vi "FirstRunTest.vi"(11 "Array":string[](array[string])) -> (2 "Message to log to console":string, 3 "exit code":i32)   [LabVIEW 2018]
uses:
  <vilib>/Utility/error.llb/DialogType.ctl
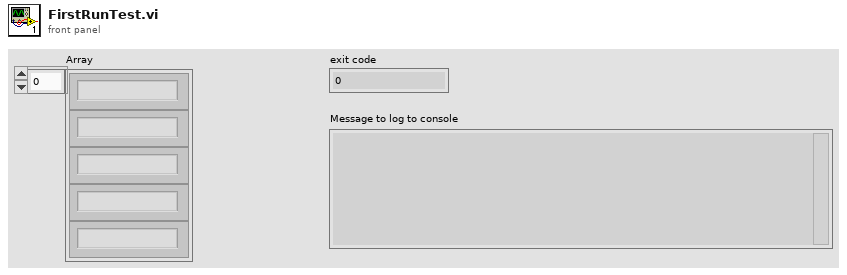
[diagram p1: front panel]
types:
  T1 = typedef "DialogType.ctl" = u16
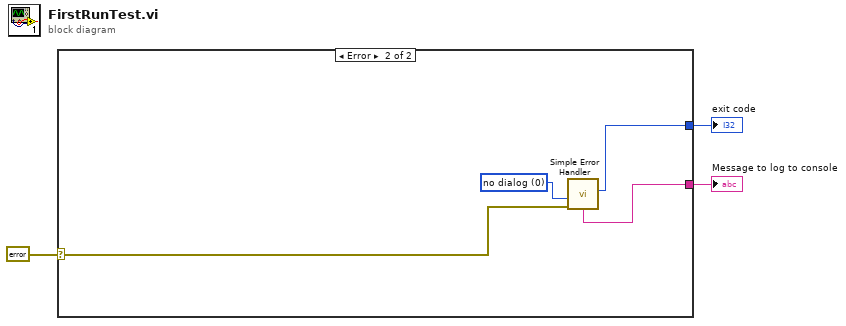
[diagram p0: block diagram]
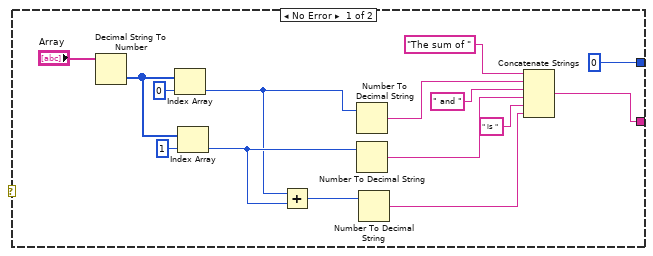
[diagram p2: hidden frame]
diagram:
  n1 = case shown="Error" errorcluster {"status"=FALSE, "code"=0, "source"=""} ("error IO") {
    selector: errorcluster {"status"=FALSE, "code"=0, "source"=""} ("error IO") -> [_ w22]
    tunnel: [0 ("exit code") w20] -> w3
    tunnel: [w4 w19] -> w2
    frame No Error {
      n2 = Decimal String To Number(string="Array") -> (number=w11:i32[])  [unwired: 2 in, 1 out]
      n3 = Index Array(array=w11, index=0) -> (element=w12:i32)
      n4 = Index Array(array=w11, index=1) -> (element=w14:i32)
      n5 = Add(x=w12, y=w14) -> (x+y=w16:i32)
      n6 = Number To Decimal String(number=w12) -> (decimal integer string=w13:string)  [unwired: 1 in]
      n7 = Number To Decimal String(number=w14) -> (decimal integer string=w15:string)  [unwired: 1 in]
      n8 = Number To Decimal String(number=w16) -> (decimal integer string=w17:string)  [unwired: 1 in]
      n9 = Concatenate Strings("The sum of " ("string"), w13, " and " ("string"), w15, " is " ("string"), w17) -> (w4:string)
    }
    frame Error {
      w21 = T1 0 items=["no dialog", "OK message", "continue or stop message", "OK message + warnings", "continue/stop + warnings"] ("type of dialog (OK msg:1)")
      n10 = call <vilib>:"Simple Error Handler.vi"("type of dialog (OK msg:1)"=w21, "error in (no error)"=w22) -> ("code out"=w20:i32, "message"=w19:string)  [unwired: 3 in, 3 out]
    }
  }
  "exit code" <- w3
  "Message to log to console" <- w2
